vi "Get imaging buffer.vi"(8 "error in (no error)":errorcluster, 11 "DAQMH121119OrcaFlash in":refnum<class "DAQOrcaFlash.lvclass">) -> (0 "error out":errorcluster, 1 "Buffer 2":u16[][](array[numeric]), 2 "imaging buffer":T1, 3 "DAQMH121119OrcaFlash out":refnum<class "DAQOrcaFlash.lvclass">, 4 "Image type":u32)   [LabVIEW 2012, in "DAQOrcaFlash.lvclass"]
uses:
  DAQOrcaFlash.lvclass
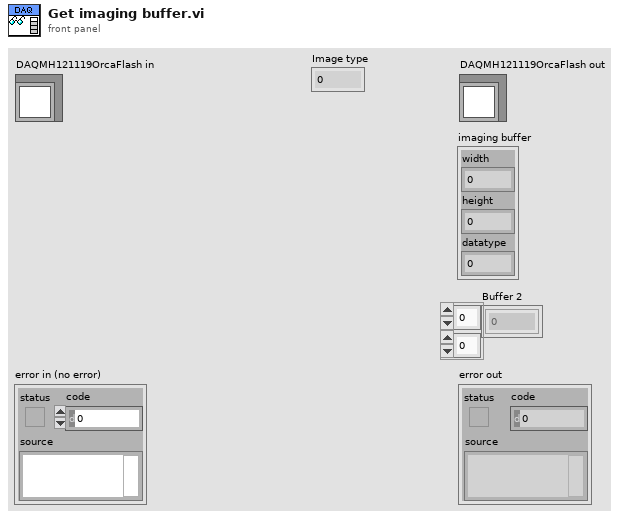
[diagram p1: front panel]
types:
  T1 = cluster{"width":u32, "height":u32, "datatype":u32}
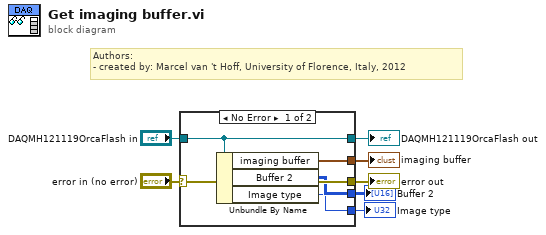
[diagram p0: block diagram]
diagram:
  # "Authors: \n- created by: Marcel van 't Hoff, University of Florence, Italy, 2012"
  n1 = case shown="No Error" "error in (no error)" {
    selector: "error in (no error)" -> [w12 w14]
    tunnel: [w12 w14] -> w6
    tunnel: [w11 w13] -> w4
    tunnel: "DAQMH121119OrcaFlash in" -> [w11 w13]
    tunnel: [w10 _] -> w3
    tunnel: [w9 _] -> w2
    tunnel: [w8 _] -> w1
    frame No Error {
      n2 = Unbundle By Name(w11) -> ("imaging buffer"=w10:T1, "Buffer 2"=w9:u16[][], "Image type"=w8:u32)
    }
    frame Error {
    }
  }
  "error out" <- w6
  "DAQMH121119OrcaFlash out" <- w4
  "imaging buffer" <- w3
  "Buffer 2" <- w2
  "Image type" <- w1
